vi "Begin.vi"(8 "error in":errorcluster) -> (0 "error out":errorcluster)   [LabVIEW 2018]
doc: "Called before other user functions, this VI can be used to open I/O refnums, load in file data, and do general program initialization. Notice that the <B>error out</B> terminal is simply used for data flow. Wiring it to other structures or subVIs ensures that this VI runs first."
uses:
  <vilib>/Rock Robotics/WPI/DriverStation/WPI_DriverStationRobotMode2.ctl
  <vilib>/Rock Robotics/WPI/Joystick/WPI_JoystickDeviceEnum.ctl
  <vilib>/Rock Robotics/WPI/SafetyOutput/WPI_SafetyOutputConfigMenu.ctl
  <vilib>/Rock Robotics/WPI/ThirdParty/Phoenix-LabVIEW/Motor Controller/Controls/CTRE_Phoenix_MotorControl_ControlMode.ctl
  <vilib>/Rock Robotics/WPI/ThirdParty/Phoenix-LabVIEW/Motor Controller/Controls/CTRE_Phoenix_MotorControl_FeedbackDevice.ctl
  <vilib>/Rock Robotics/WPI/ThirdParty/Phoenix-LabVIEW/Motor Controller/Controls/CTRE_Phoenix_MotorControl_NeutralMode.ctl
  <vilib>/Rock Robotics/SystemInterfaces/AI/FPGA_AIChannel.ctl
  <vilib>/Rock Robotics/WPI/Solenoid/WPI_SolenoidChannel.ctl
  Robot Global Data.vi
  <vilib>/Rock Robotics/Network Tables/NT Write String Array.vi
  <vilib>/Rock Robotics/WPI/RobotDrive/WPI_RobotDriveOpen4MotorWithExistingMotors.vi
  <vilib>/Rock Robotics/WPI/Switch/WPI_SwitchOpenLimit.vi
  <vilib>/Rock Robotics/WPI/Ultrasonic/WPI_SonarMB1010AnalogOpen.vi
  <vilib>/Rock Robotics/WPI/Ultrasonic/WPI_SonarMB1010AnalogRefNum Registry Set.vi
  <vilib>/Rock Robotics/WPI/Solenoid/WPI_SolenoidOpenDouble.vi
  <vilib>/Rock Robotics/WPI/Utilities/WPI_GetSetVariantRefNum.vi
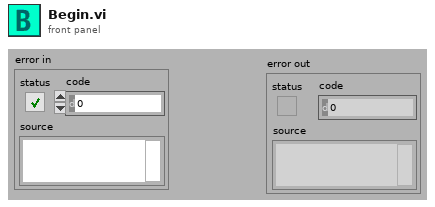
[diagram p1: front panel]
types:
  T1 = typedef "WPI_SolenoidChannel.ctl" = enum8{"Solenoid 0", "Solenoid 1", "Solenoid 2", "Solenoid 3", "Solenoid 4", "Solenoid 5", "Solenoid 6", "Solenoid 7", "Invalid"}
  T2 = typedef "WPI_JoystickDeviceEnum.ctl" = enum16{"USB 0", "USB 1", "USB 2", "USB 3", "USB 4", "USB 5"}
  T3 = typedef "FPGA_AIChannel.ctl" = enum8{"AI 0", "AI 1", "AI 2", "AI 3", "AI MXP 0", "AI MXP 1", "AI MXP 2", "AI MXP 3", "Invalid"}
  T4 = typedef "CTRE_Phoenix_MotorControl_FeedbackDevice.ctl" = i8
  T5 = typedef "CTRE_Phoenix_MotorControl_NeutralMode.ctl" = enum8{"EEPROMSetting", "Override to Coast", "Override to Brake"}
  T6 = typedef "CTRE_Phoenix_MotorControl_ControlMode.ctl" = u16
  T7 = typedef "WPI_SafetyOutputConfigMenu.ctl" = enum16{"Enable", "Disable"}
  T8 = typedef "WPI_DriverStationRobotMode2.ctl" = enum16{"Autonomous Disabled", "Autonomous Enabled", "Teleop Disabled", "Teleop Enabled", "Disconnected", "Finish", "Test Disabled", "Test Enabled", "Emergency Stopped"}
  T9 = typedef "WPI_MotorControlDeviceRef.ctl" = cluster{"DeviceStatus":errorcluster, "Type":T10, "PWM":cluster{"PWM Channel":T11, "DeadBand":T12}, "CAN":cluster{"Device Number":u8, "SetOutput VI Ref":variant, "GetOutput VI Ref":variant, "Enable VI Ref":variant, "Disable VI Ref":variant, "Data":variant}, "Invert":bool, "DIO PWM":cluster{"PWM \"Enable\" Channel":T11, "DIOChannel":T13, "PWM Rate":dbl}}
  T10 = typedef "WPI_MotorControlType.ctl" = enum16{"PWM", "CAN", "DIO PWM"}
  T11 = typedef "FPGA_DIOPWMChannel.ctl" = enum8{"PWM 0", "PWM 1", "PWM 2", "PWM 3", "PWM 4", "PWM 5", "PWM 6", "PWM 7", "PWM 8", "PWM 9", "PWM MXP 0", "PWM MXP 1", "PWM MXP 2", "PWM MXP 3", "PWM MXP 4", "PWM MXP 5", "PWM MXP 6", "PWM MXP 7", "PWM MXP 8", "PWM MXP 9", "Invalid"}
  T12 = typedef "WPI_PWMDeadband.ctl" = cluster{"Name":string, "maxPositivePwm":i32, "minPositivePwm":i32, "centerPwm":i32, "maxNegativePwm":i32, "minNegativePwm":i32, "angularRange":u16}
  T13 = typedef "FPGA_DIOChannel.ctl" = enum8{"DIO 0", "DIO 1", "DIO 2", "DIO 3", "DIO 4", "DIO 5", "DIO 6", "DIO 7", "DIO 8", "DIO 9", "DIO MXP 0", "DIO MXP 1", "DIO MXP 2", "DIO MXP 3", "DIO MXP 4", "DIO MXP 5", "DIO MXP 6", "DIO MXP 7", "DIO MXP 8", "DIO MXP 9", "DIO MXP 10", "DIO MXP 11", "DIO MXP 12", "DIO MXP 13", "DIO MXP 14", "DIO MXP 15", "SPI Port CS1", "SPI Port CS2", "SPI Port CS3", "SPI Port MISO", "SPI Port MOSI", "Invalid"}
  T14 = typedef "WPI_SwitchDevRef.ctl" = cluster{"DevStatus":errorcluster, "DIO Channel":T13, "CntIndex":T15, "Normally Closed":bool}
  T15 = typedef "FPGA_CounterCtrSystemIndex.ctl" = enum8{"Ctr 0", "Ctr 1", "Ctr 2", "Ctr 3", "Ctr 4", "Ctr 5", "Ctr 6", "Ctr 7", "Invalid"}
  T16 = typedef "WPI_JoystickDevRef.ctl" = cluster{"Device":T2}
  T17 = typedef "WPI_SolenoidDevRef.ctl" = cluster{"DevStatus":errorcluster, "Pneumatics Control Module":u8, "Forward Solenoid Channel":T1, "Reverse Solenoid Channel":T1}
  T18 = typedef "WPI_CompressorDevRef.ctl" = cluster{"DevStatus":errorcluster, "Pneumatics Control Module":u8}
  T19 = typedef "WPI_SonarMB1010AnalogDeviceRef.ctl" = cluster{"AIDeviceRef":T20, "Scaling factor (V/in)":dbl, "Average Bits":u8}
  T20 = typedef "WPI_AnalogChannelDevRef.ctl" = cluster{"DevStatus":errorcluster, "Analog Channel":T3}
  T21 = typedef "WPI_RobotDriveDevRef.ctl" = cluster{"DevStatus":errorcluster, "Motors[]":T9[], "Square Inputs":bool, "Max Output":dbl}
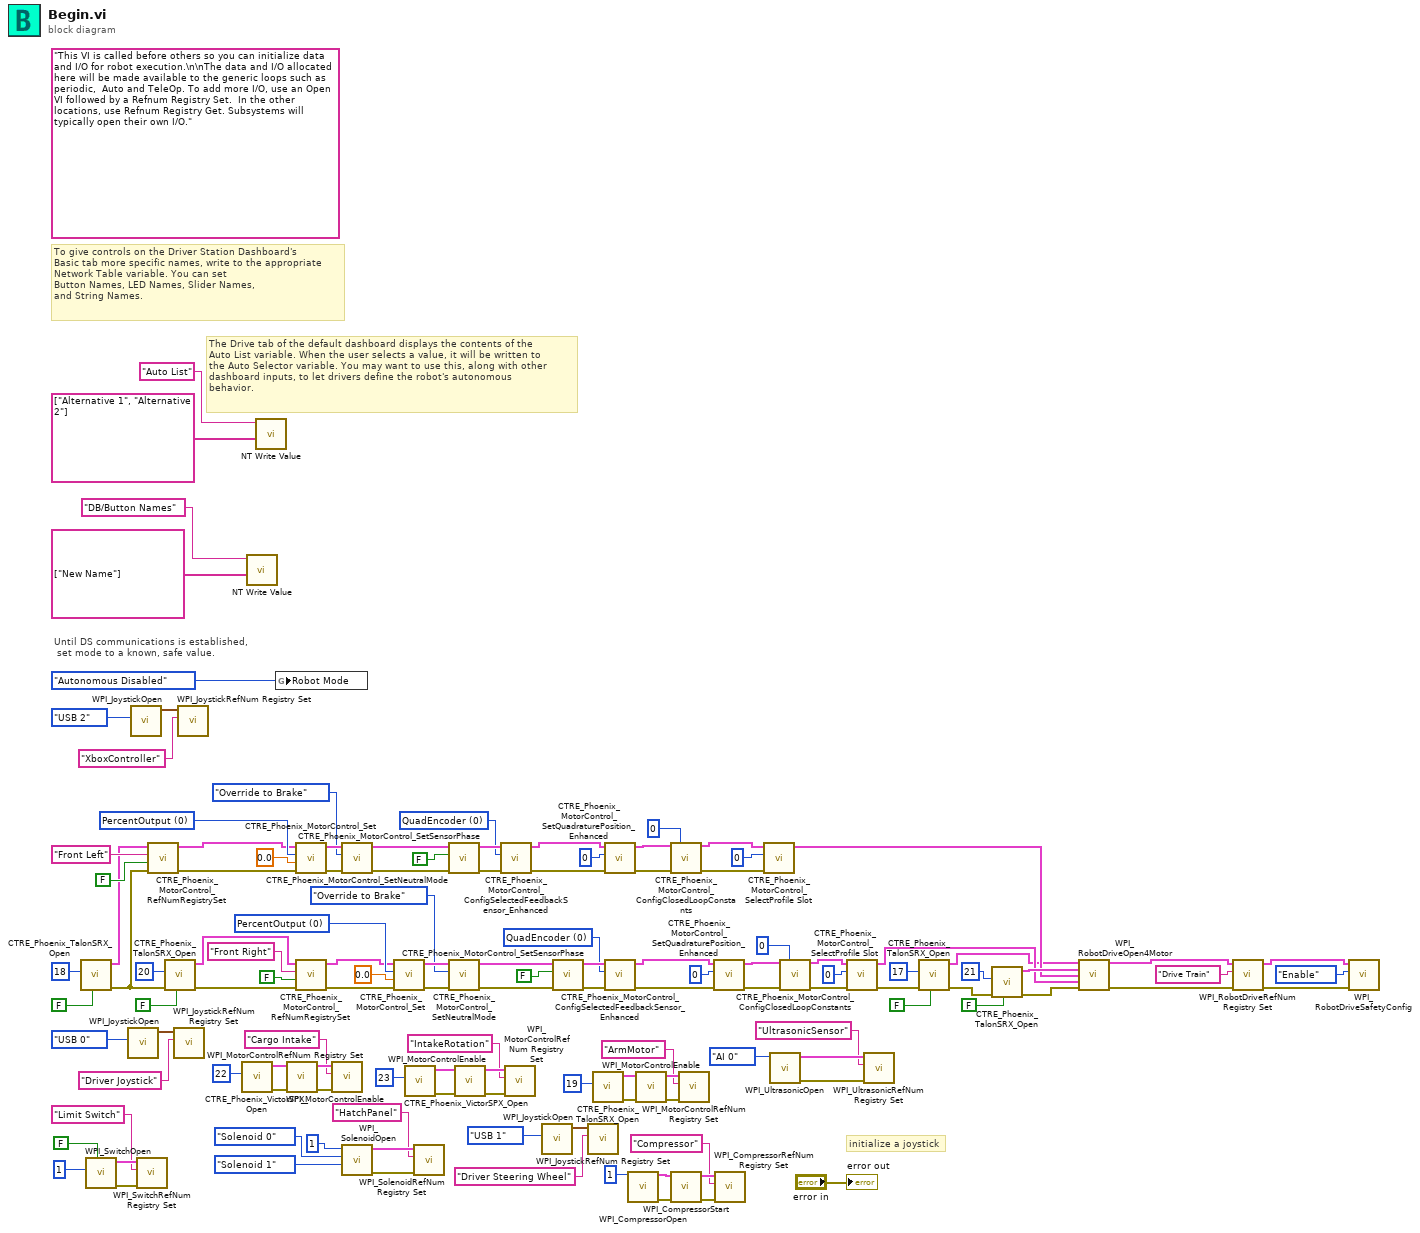
[diagram p0: block diagram]
diagram:
  w60 = T4 0 items=["None"=-1, "QuadEncoder"=0, "Analog"=2, "Tachometer"=4, "Pulse Width Encoded Position"=8, "Sensor Sum (S0 + S1)"=9, "Sensor Difference (D0 - D1)"=10, "Remote Source 0"=11, "Remote Source 1"=12, "Software Emulated"=15] ("Feedback Device")
  w49 = T6 0 items=["PercentOutput"=0, "Position"=1, "Velocity"=2, "Current"=3, "Follower"=5, "MotionProfile"=6, "MotionMagic"=7, "MotionMagicArc"=8, "MotionProfileArc"=10, "Disabled"=15] ("Control Mode")
  w88 = T4 0 items=["None"=-1, "QuadEncoder"=0, "Analog"=2, "Tachometer"=4, "Pulse Width Encoded Position"=8, "Sensor Sum (S0 + S1)"=9, "Sensor Difference (D0 - D1)"=10, "Remote Source 0"=11, "Remote Source 1"=12, "Software Emulated"=15] ("Feedback Device")
  w77 = T6 0 items=["PercentOutput"=0, "Position"=1, "Velocity"=2, "Current"=3, "Follower"=5, "MotionProfile"=6, "MotionMagic"=7, "MotionMagicArc"=8, "MotionProfileArc"=10, "Disabled"=15] ("Control Mode")
  (unwired) "This VI is called before others so you can initialize data and I/O for robot execution.\n\nThe data and I/O allocated here will be made available to the generic loops such as periodic,  Auto and TeleOp. To add more I/O, use an Open VI followed by a Refnum Registry Set.  In the other locations, use Refnum Registry Get. Subsystems will typically open their own I/O."
  # "The Drive tab of the default dashboard displays the contents of the\nAuto List variable. When the user selects a value, it will be written to\nthe Auto Selector variable. You may want to use this, along with other\ndashboard inputs, to let drivers define the robot's autonomous\nbehavior."
  # "To give controls on the Driver Station Dashboard's\nBasic tab more specific names, write to the appropriate\nNetwork Table variable. You can set\nButton Names, LED Names, Slider Names,\nand String Names."
  # "initialize a joystick"
  # "Until DS communications is established,\n set mode to a known, safe value."
  n1 = call <vilib>:"CTRE_Phoenix_TalonSRX_Open.vi"("Invert"=FALSE, "Device Number"=u8 18) -> ("error out"=w23:errorcluster, "CAN Talon SRX Ref"=w69:T9)  [unwired: 8 in]
  n2 = call-poly <vilib>:"WPI_SwitchOpen.vi"("Normally Closed"=FALSE, "DIO Channel"=1) -> ("error out"=w35:errorcluster, "SwitchDevRef"=w38:T14)  [unwired: 8 in]
  n3 = call <vilib>:"WPI_JoystickOpen.vi"("JoystickDevice"=WPI_JoystickDeviceEnum."USB 0") -> ("JoystickDevRef"=w125:T16)  [unwired: 10 in]
  n4 = call <vilib>:"WPI_JoystickOpen.vi"("JoystickDevice"=WPI_JoystickDeviceEnum."USB 2") -> ("JoystickDevRef"=w25:T16)  [unwired: 10 in]
  n5 = call <vilib>:"WPI_SwitchRefNum Registry Set.vi"("error in (no error)"=w35, "refnum name"="Limit Switch", "SwitchDevRef"=w38) -> ()  [unwired: 7 in, 2 out]
  n6 = call <vilib>:"CTRE_Phoenix_MotorControl_RefNumRegistrySet.vi"("error in (no error)"=w23, "Test Mode Only"=FALSE, "refnum name"="Front Left", "PhoenixMotorControlDevRef"=w69) -> ("error out"=w47:errorcluster, "PhoenixMotorControlDevRef"=w48:T9)  [unwired: 6 in]
  n7 = call <vilib>:"CTRE_Phoenix_TalonSRX_Open.vi"("Invert"=FALSE, "error in"=w23, "Device Number"=u8 20) -> ("error out"=w97:errorcluster, "CAN Talon SRX Ref"=w98:T9)  [unwired: 7 in]
  n8 = call <vilib>:"WPI_JoystickRefNum Registry Set.vi"("refnum name"="Driver Joystick", "JoystickDevRef"=w125) -> ()  [unwired: 8 in, 2 out]
  n9 = call <vilib>:"WPI_JoystickRefNum Registry Set.vi"("refnum name"="XboxController", "JoystickDevRef"=w25) -> ()  [unwired: 8 in, 2 out]
  n10 = call <vilib>:"CTRE_Phoenix_VictorSPX_Open.vi"("Device Number"=22) -> ("error out"=w44:errorcluster, "CAN Talon SRX Ref"=w43:T9)  [unwired: 9 in]
  n11 = call-poly <vilib>:"NT Write Value.vi"("String Array"=string[] ["New Name"], "Name"="DB/Button Names") -> ()  [unwired: 9 in, 1 out]
  n12 = call-poly <vilib>:"NT Write Value.vi"("String Array"=string[] ["Alternative 1", "Alternative 2"], "Name"="Auto List") -> ()  [unwired: 9 in, 1 out]
  n13 = global write "Robot Global Data.vi" "Robot Mode"(WPI_DriverStationRobotMode2."Autonomous Disabled" ("Robot Mode")) -> ()
  n14 = call <vilib>:"WPI_MotorControlEnable.vi"("error in (no error)"=w44, "CAN MotorDevRef"=w43) -> ("error out"=w104:errorcluster, "CAN MotorDevRef"=w103:T9)  [unwired: 8 in]
  n15 = call <vilib>:"CTRE_Phoenix_MotorControl_Set.vi"("error in (no error)"=w47, "Output"=0.0, "Control Mode"=w49, "PhoenixMotorControlDevRef"=w48) -> ("error out"=w64:errorcluster, "PhoenixMotorControlDevRef"=w68:T9)  [unwired: 6 in]
  n16 = call <vilib>:"CTRE_Phoenix_MotorControl_RefNumRegistrySet.vi"("error in (no error)"=w97, "Test Mode Only"=FALSE, "refnum name"="Front Right", "PhoenixMotorControlDevRef"=w98) -> ("error out"=w75:errorcluster, "PhoenixMotorControlDevRef"=w76:T9)  [unwired: 6 in]
  n17 = call <vilib>:"WPI_MotorControlRefNum Registry Set.vi"("error in (no error)"=w104, "refnum name"="Cargo Intake", "MotorControlDevRef"=w103) -> ()  [unwired: 7 in, 2 out]
  n18 = call <vilib>:"CTRE_Phoenix_MotorControl_SetNeutralMode.vi"("error in (no error)"=w64, "Motor Control Neutral Mode"=CTRE_Phoenix_MotorControl_NeutralMode."Override to Brake", "PhoenixMotorControlDevRef"=w68) -> ("error out"=w66:errorcluster, "PhoenixMotorControlDevRef"=w65:T9)  [unwired: 7 in]
  n19 = call-poly <vilib>:"WPI_SolenoidOpen.vi"("Reverse Solenoid Channel"=WPI_SolenoidChannel."Solenoid 1", "Forward Solenoid Channel"=WPI_SolenoidChannel."Solenoid 0", "Pneumatics Control Module (0)"=u8 1) -> ("error out"=w9:errorcluster, "SolenoidDevRef"=w10:T17)  [unwired: 7 in]
  n20 = call <vilib>:"CTRE_Phoenix_MotorControl_Set.vi"("error in (no error)"=w75, "Output"=0.0, "Control Mode"=w77, "PhoenixMotorControlDevRef"=w76) -> ("error out"=w92:errorcluster, "PhoenixMotorControlDevRef"=w96:T9)  [unwired: 6 in]
  n21 = call <vilib>:"CTRE_Phoenix_VictorSPX_Open.vi"("Device Number"=23) -> ("error out"=w15:errorcluster, "CAN Talon SRX Ref"=w16:T9)  [unwired: 9 in]
  n22 = call <vilib>:"WPI_SolenoidRefNum Registry Set.vi"("error in (no error)"=w9, "refnum name"="HatchPanel", "SolenoidDevRef"=w10) -> ()  [unwired: 7 in, 2 out]
  n23 = call <vilib>:"CTRE_Phoenix_MotorControl_SetSensorPhase.vi"("error in (no error)"=w66, "PhaseSensor"=FALSE, "PhoenixMotorControlDevRef"=w65) -> ("error out"=w62:errorcluster, "PhoenixMotorControlDevRef"=w61:T9)  [unwired: 7 in]
  n24 = call <vilib>:"CTRE_Phoenix_MotorControl_SetNeutralMode.vi"("error in (no error)"=w92, "Motor Control Neutral Mode"=CTRE_Phoenix_MotorControl_NeutralMode."Override to Brake", "PhoenixMotorControlDevRef"=w96) -> ("error out"=w94:errorcluster, "PhoenixMotorControlDevRef"=w93:T9)  [unwired: 7 in]
  n25 = call <vilib>:"WPI_MotorControlEnable.vi"("error in (no error)"=w15, "CAN MotorDevRef"=w16) -> ("error out"=w19:errorcluster, "CAN MotorDevRef"=w18:T9)  [unwired: 8 in]
  n26 = call <vilib>:"CTRE_Phoenix_MotorControl_ConfigSelectedFeedbackSensor_Enhanced.vi"("error in (no error)"=w62, "Feedback Device"=w60, "PhoenixMotorControlDevRef"=w61) -> ("error out"=w58:errorcluster, "PhoenixMotorControlDevRef"=w59:T9)  [unwired: 7 in]
  n27 = call <vilib>:"WPI_MotorControlRefNum Registry Set.vi"("error in (no error)"=w19, "refnum name"="IntakeRotation", "MotorControlDevRef"=w18) -> ()  [unwired: 7 in, 2 out]
  n28 = call <vilib>:"WPI_JoystickOpen.vi"("JoystickDevice"=WPI_JoystickDeviceEnum."USB 1") -> ("JoystickDevRef"=w106:T16)  [unwired: 10 in]
  n29 = call <vilib>:"CTRE_Phoenix_MotorControl_SetSensorPhase.vi"("error in (no error)"=w94, "PhaseSensor"=FALSE, "PhoenixMotorControlDevRef"=w93) -> ("error out"=w90:errorcluster, "PhoenixMotorControlDevRef"=w89:T9)  [unwired: 7 in]
  n30 = call <vilib>:"WPI_JoystickRefNum Registry Set.vi"("refnum name"="Driver Steering Wheel", "JoystickDevRef"=w106) -> ()  [unwired: 8 in, 2 out]
  n31 = call <vilib>:"CTRE_Phoenix_TalonSRX_Open.vi"("Device Number"=19) -> ("error out"=w31:errorcluster, "CAN Talon SRX Ref"=w30:T9)  [unwired: 9 in]
  n32 = call <vilib>:"CTRE_Phoenix_MotorControl_SetQuadraturePosition_Enhanced.vi"("error in (no error)"=w58, "New Position"=0, "PhoenixMotorControlDevRef"=w59) -> ("error out"=w55:errorcluster, "PhoenixMotorControlDevRef"=w56:T9)  [unwired: 7 in]
  n33 = call <vilib>:"CTRE_Phoenix_MotorControl_ConfigSelectedFeedbackSensor_Enhanced.vi"("error in (no error)"=w90, "Feedback Device"=w88, "PhoenixMotorControlDevRef"=w89) -> ("error out"=w86:errorcluster, "PhoenixMotorControlDevRef"=w87:T9)  [unwired: 7 in]
  n34 = call <vilib>:"WPI_CompressorOpen.vi"("Pneumatics Control Module (0)"=u8 1) -> ("CompressorDevRef"=w6:T18, "error out"=w7:errorcluster)  [unwired: 13 in]
  n35 = call <vilib>:"WPI_MotorControlEnable.vi"("error in (no error)"=w31, "CAN MotorDevRef"=w30) -> ("error out"=w29:errorcluster, "CAN MotorDevRef"=w28:T9)  [unwired: 8 in]
  n36 = call <vilib>:"CTRE_Phoenix_MotorControl_ConfigClosedLoopConstants.vi"("PhoenixMotorControlDevRef"=w56, "slotIdx"=0, "error in (no error)"=w55) -> ("PhoenixMotorControlDevRef"=w52:T9, "error out"=w53:errorcluster)  [unwired: 11 in]
  n37 = call <vilib>:"WPI_CompressorStart.vi"("error in (no error)"=w7, "CompressorDevRef"=w6) -> ("error out"=w4:errorcluster, "CompressorDevRef"=w5:T18)  [unwired: 8 in]
  n38 = call <vilib>:"WPI_MotorControlRefNum Registry Set.vi"("error in (no error)"=w29, "refnum name"="ArmMotor", "MotorControlDevRef"=w28) -> ()  [unwired: 7 in, 2 out]
  n39 = call <vilib>:"CTRE_Phoenix_MotorControl_SetQuadraturePosition_Enhanced.vi"("error in (no error)"=w86, "New Position"=0, "PhoenixMotorControlDevRef"=w87) -> ("error out"=w83:errorcluster, "PhoenixMotorControlDevRef"=w84:T9)  [unwired: 7 in]
  n40 = call <vilib>:"WPI_CompressorRefNum Registry Set.vi"("error in (no error)"=w4, "refnum name"="Compressor", "CompressorDevRef"=w5) -> ()  [unwired: 7 in, 2 out]
  n41 = call <vilib>:"CTRE_Phoenix_MotorControl_SelectProfile Slot.vi"("error in (no error)"=w53, "slotIdx"=0, "PhoenixMotorControlDevRef"=w52) -> ("PhoenixMotorControlDevRef"=w45:T9)  [unwired: 7 in, 1 out]
  n42 = call-poly <vilib>:"WPI_UltrasonicOpen.vi"("Analog Channel"=FPGA_AIChannel."AI 0") -> ("error out"=w41:errorcluster, "SonarMB1010AnalogDevRef"=w40:T19)  [unwired: 9 in]
  n43 = call <vilib>:"CTRE_Phoenix_MotorControl_ConfigClosedLoopConstants.vi"("PhoenixMotorControlDevRef"=w84, "slotIdx"=0, "error in (no error)"=w83) -> ("PhoenixMotorControlDevRef"=w80:T9, "error out"=w81:errorcluster)  [unwired: 11 in]
  n44 = call <vilib>:"CTRE_Phoenix_MotorControl_SelectProfile Slot.vi"("error in (no error)"=w81, "slotIdx"=0, "PhoenixMotorControlDevRef"=w80) -> ("error out"=w22:errorcluster, "PhoenixMotorControlDevRef"=w73:T9)  [unwired: 7 in]
  n45 = call-poly <vilib>:"WPI_UltrasonicRefNum Registry Set.vi"("error in (no error)"=w41, "refnum name"="UltrasonicSensor", "SonarMB1010AnalogDevRef"=w40) -> ()  [unwired: 7 in, 2 out]
  n46 = call <vilib>:"CTRE_Phoenix_TalonSRX_Open.vi"("Invert"=FALSE, "error in"=w22, "Device Number"=17) -> ("error out"=w21:errorcluster, "CAN Talon SRX Ref"=w1:T9)  [unwired: 7 in]
  n47 = call <vilib>:"CTRE_Phoenix_TalonSRX_Open.vi"("Invert"=FALSE, "error in"=w21, "Device Number"=21) -> ("error out"=w20:errorcluster, "CAN Talon SRX Ref"=w118:T9)  [unwired: 7 in]
  n48 = call-poly <vilib>:"WPI_RobotDriveOpen4Motor.vi"("Rear Left Motor Dev Ref"=w1, "Rear Right Motor Dev Ref"=w118, "Front Left Motor Dev Ref"=w45, "Front Right Motor Dev Ref"=w73, "error in (no error)"=w20) -> ("RobotDriveDevRef"=w117:T21, "error out"=w116:errorcluster)  [unwired: 9 in]
  n49 = call <vilib>:"WPI_RobotDriveRefNum Registry Set.vi"("error in (no error)"=w116, "refnum name"="Drive Train", "RobotDriveDevRef"=w117) -> ("error out"=w109:errorcluster, "RobotDriveDevRef"=w110:T21)  [unwired: 7 in]
  n50 = call <vilib>:"WPI_RobotDriveSafetyConfig.vi"("error in (no error)"=w109, "mode"=WPI_SafetyOutputConfigMenu."Enable", "RobotDriveDevRef"=w110) -> ()  [unwired: 7 in, 2 out]
  "error out" <- "error in"
